vi "Nascondi colonne.vi"(9 "LINGUA":i32, 10 "TIPO COLLEGAMENTO":u16, 11 "Array":refnum<vi>[](array[refnum])) -> (0 "decimali":i32[][](array[numeric]))   [LabVIEW 2019]
uses:
  Global percorso impostazioni.vi
  <vilib>/Utility/file.llb/Read Delimited Spreadsheet (string).vi
panel:
  out "x = y?":bool
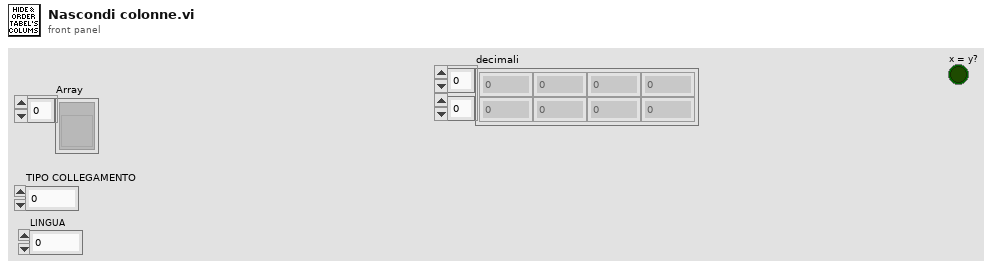
[diagram p1: front panel]
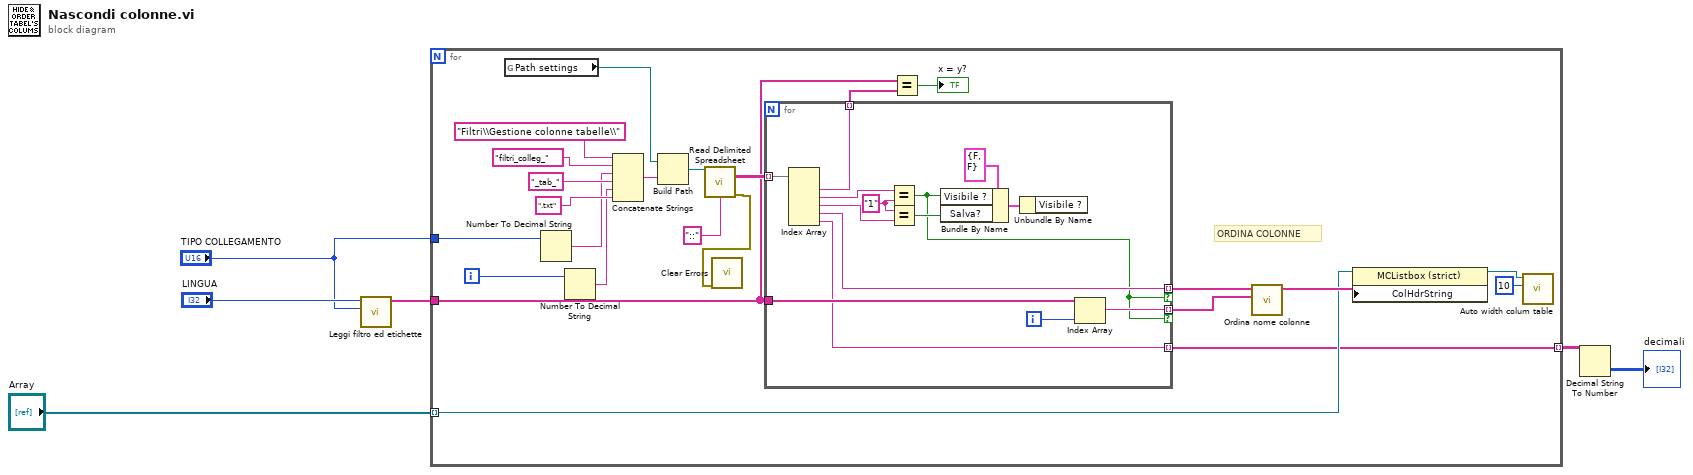
[diagram p0: block diagram]
diagram:
  n1 = call "Leggi filtro ed etichette.vi"("ID COLLEGAMENTO"="TIPO COLLEGAMENTO", "LINGUA"="LINGUA") -> ("ETICHETTE"=w5:string[])  [unwired: 4 in, 5 out]
  n2 = for {
    tunnel: "Array" -> [w18] mode=indexing
    tunnel: w5 -> [w10]
    tunnel: "TIPO COLLEGAMENTO" -> [w17]
    tunnel: [w14] -> w1 mode=indexing
    i -> [w7]
    # "ORDINA COLONNE"
    n3 = global read "Global percorso impostazioni.vi" "Path settings"() -> (w24:path)
    n4 = Number To Decimal String(number=w17) -> (decimal integer string=w13:string)  [unwired: 1 in]
    n5 = Number To Decimal String(number=w7) -> (decimal integer string=w12:string)  [unwired: 1 in]
    n6 = Concatenate Strings("Filtri\\Gestione colonne tabelle\\" ("name or relative path"), "filtri_colleg_" ("string"), w13, "_tab_" ("string"), w12, ".txt" ("string")) -> (w25:string)
    n7 = Build Path(base path=w24, name or relative path=w25) -> (appended path=w19:path)
    n8 = call-poly <vilib>:"Read Delimited Spreadsheet.vi"("file path (dialog if empty)"=w19, "delimiter (\\t)"="::" ("delimiter (\\t)")) -> ("all rows"=w30:string[][], "error out"=w8:errorcluster)  [unwired: 8 in, 4 out]
    n9 = call <vilib>:"Clear Errors.vi"("error in (no error)"=w8) -> ()  [unwired: 5 in, 2 out]
    n10 = for {
      tunnel: w30 -> [w44] mode=indexing
      tunnel: [w37] -> w27 mode=indexing if=w32
      tunnel: w10 -> [w36]
      tunnel: [w34] -> w28 mode=indexing if=w32
      tunnel: [w33] -> w14 mode=indexing
      tunnel: [w31] -> w11 mode=indexing
      i -> [w38]
      w40 = "1" ("y")
      n11 = Index Array(array=w44) -> (element #1=w31:string, element #2=w43:string, element #3=w41:string, element #4=w34:string, element #5=w33:string)  [unwired: 5 in]
      n12 = Equal?(x=w43, y=w40) -> (x = y?=w32:bool)
      n13 = Equal?(x=w40, y=w41) -> (x = y?=w42:bool)
      n14 = Bundle By Name(cluster=cluster{"Visibile ?":bool, "Salva?":bool} {"Visibile ?"=FALSE, "Salva?"=FALSE} ("QH"), "Visibile ?"=w32, "Salva?"=w42) -> (w35:cluster{"Visibile ?":bool, "Salva?":bool})
      n15 = Unbundle By Name(w35) -> ()  [unwired: 1 out]
      n16 = Index Array(array=w36, index=w38) -> (element=w37:string)
    }
    n17 = Equal?(x=w10, y=w11) -> (x = y?=→"x = y?":bool)
    n18 = call "Ordina nome colonne.vi"("Array nomi"=w27, "Array indici"=w28) -> ("Array nomi ordinati"=w26:string[])  [unwired: 9 in]
    n19 = property class="MCListbox (strict)"(reference=w18, "ColHdrString"=w26) -> (reference out=w15:refnum<vi>)  [unwired: 1 in, 1 out]
    n20 = call "Auto width colum table.vi"("spazi"=i16 10, "Real Time tabella"=w15) -> ()  [unwired: 9 in, 1 out]
  }
  n21 = Decimal String To Number(string=w1) -> (number=→"decimali":i32[][])  [unwired: 2 in, 1 out]
